vi "U16转浮点ABCD.vi"(11 "U16":u16[](array[numeric]) format="%x") -> (3 "Float ABCD":sgl[](array[numeric]))   [LabVIEW 2016, in "WL-1A1.lvlib"]
uses:
  WL-1A1.lvlib
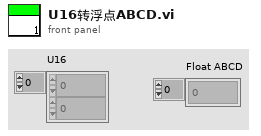
[diagram p1: front panel]
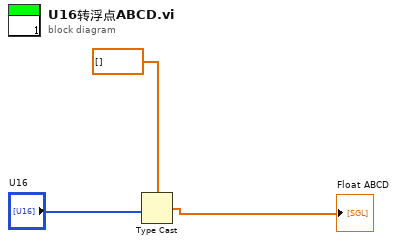
[diagram p0: block diagram]
diagram:
  n1 = Type Cast(type=sgl[] [], x="U16") -> (*(type *) &x=→"Float ABCD":sgl[])
